vi "UpdateFPReply.vi"(2 "success?":bool, 3 "Reply":string, 4 "Sent":string, 5 "method":string) -> ()   [LabVIEW 2013]
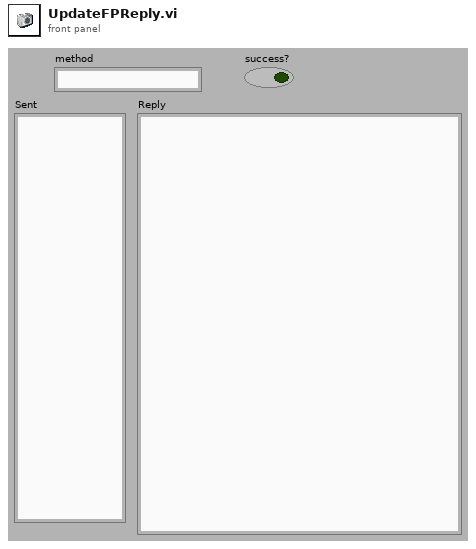
[diagram p1: front panel]
types:
  T1 = cluster{"Sent":string, "Reply":string, "method":string, "success?":bool, "element":string, "element":string, "Current Time":string}
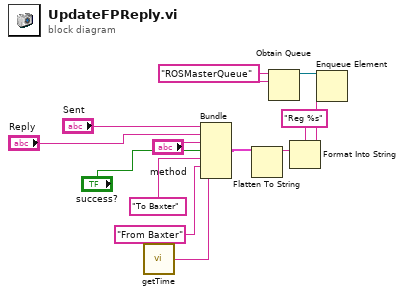
[diagram p0: block diagram]
diagram:
  w4 = "ROSMasterQueue" ("name (unnamed)")
  n1 = call "getTime.vi"() -> ("Current Time"=w1:string)  [unwired: 1 in]
  n2 = Bundle("Sent"="Sent", "Reply"="Reply", "method"="method", "success?"="success?", "element"="To Baxter", "element"="From Baxter", "Current Time"=w1) -> (w11:T1)  [unwired: 1 in]
  n3 = Flatten To String(anything=w11) -> (data string=w12:string)  [unwired: 3 in, 2 out]
  n4 = Obtain Queue(name (unnamed)=w4, element data type=w4) -> (queue out=w5:refnum<queue>)  [unwired: 3 in, 2 out]
  n5 = Format Into String(format string="Reg %s" ("element"), w12) -> (resulting string=w13:string)  [unwired: 2 in, 1 out]
  n6 = Enqueue Element(queue=w5, element=w13) -> ()  [unwired: 2 in, 3 out]
